vi "Data2Stats.vi"(0 "CMD Step":dbl format="%#_13g", 7 "DataIn":string[][](array[string]), 11 "DesiredParameters":T1) -> (8 "StatsOut":string[][](array[string]))   [LabVIEW 2013]
uses:
  TypeDef/Command Cluster.ctl
  <vilib>/Analysis/NI_AALBase.lvlib
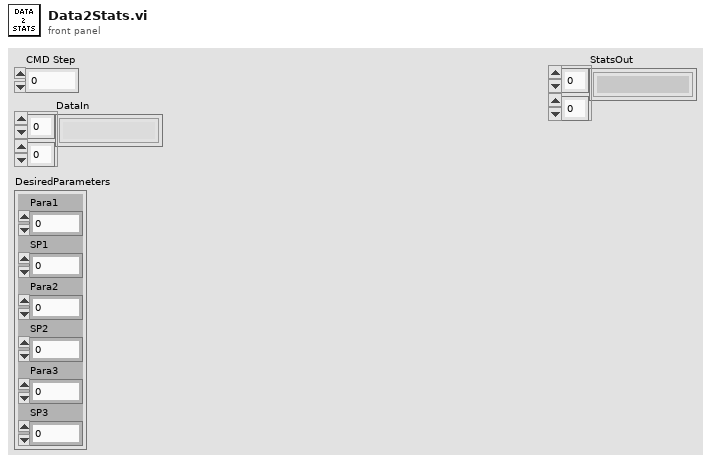
[diagram p1: front panel]
types:
  T1 = typedef "Command Cluster.ctl" = cluster{"Para1":i32, "SP1":dbl, "Para2":i32, "SP2":dbl, "Para3":i32, "SP3":dbl}
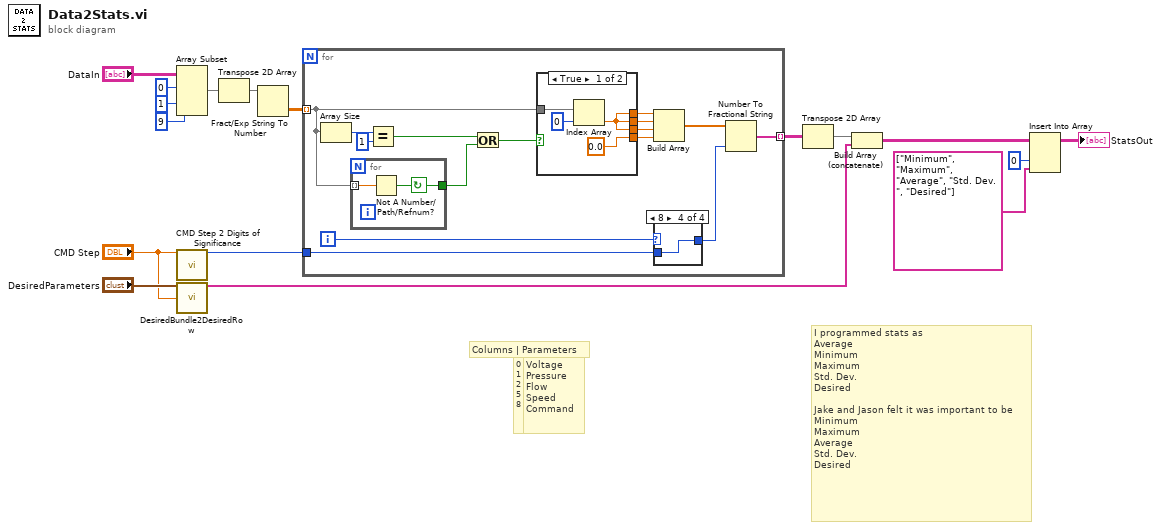
[diagram p0: block diagram]
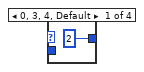
[diagram p2: hidden frame]
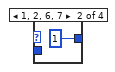
[diagram p3: hidden frame]
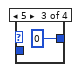
[diagram p4: hidden frame]
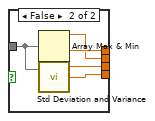
[diagram p5: hidden frame]
diagram:
  # "I programmed stats as\nAverage\nMinimum\nMaximum\nStd. Dev.\nDesired\n\nJake and Jason felt it was important to be\nMinimum\nMaximum\nAverage\nStd. Dev.\nDesired"
  # "Columns | Parameters"
  # "0\n1\n2\n5\n8"
  # "Voltage\nPressure\nFlow\nSpeed\nCommand"
  n1 = Array Subset(array="DataIn", index (row)=0 ("index"), index (col)=1 ("index"), length (col)=9 ("length")) -> (w13:string[][])  [unwired: 1 in]
  n2 = call "CMD Step 2 Digits of Significance.vi"("CMD Step"="CMD Step") -> ("Digits of Significance"=w2:i32)  [unwired: 14 in]
  n3 = call "DesiredBundle2DesiredRow.vi"("DesiredParameters"="DesiredParameters", "CMD Step"="CMD Step") -> ("DesiredStatRow"=w3:string[])  [unwired: 13 in]
  n4 = Transpose 2D Array(2D array=w13) -> (transposed array=w12:string[][])
  n5 = Fract/Exp String To Number(string=w12) -> (number=w11:dbl[][])  [unwired: 3 in, 1 out]
  n6 = for {
    tunnel: w11 -> [w21] mode=indexing
    tunnel: [w25] -> w5 mode=indexing
    tunnel: w2 -> [w22]
    i -> [w23]
    n7 = Array Size(array=w21) -> (size(s)=w28:i32)
    n8 = for {
      tunnel: w21 -> [w34] mode=indexing
      tunnel: [w33] -> w20
      stop <- w33 continue-if-true
      n9 = Not A Number/Path/Refnum?(number/path/refnum=w34) -> (NaN/Path/Refnum?=w33:bool)
    }
    n10 = Equal?(x=w28, y=1) -> (x = y?=w19:bool)
    n11 = Or(x=w19, y=w20) -> (x .or. y?=w18:bool)
    n12 = case shown="True" w18 {
      tunnel: [w40 w45] -> w32
      tunnel: [w40 w44] -> w31
      tunnel: [w40 w43] -> w30
      tunnel: [0.0 ("standard deviation") w47] -> w29
      tunnel: w21 -> [w42 w46]
      frame True {
        n13 = Index Array(array=w42, index=0) -> (element=w40:dbl)
      }
      frame False {
        n14 = Array Max & Min(array=w46) -> (max value=w44:dbl, min value=w45:dbl)  [unwired: 2 out]
        n15 = call <vilib>:"Std Deviation and Variance.vi"("X"=w46) -> ("mean"=w43:dbl, "standard deviation"=w47:dbl)  [unwired: 1 in, 1 out]
      }
    }
    n16 = Build Array(w32, w31, w30, w29) -> (w26:dbl[])
    n17 = case shown="8" w23 {
      tunnel: [2 1 0 w38] -> w24
      tunnel: w22 -> [_ _ _ w38]
      frame 0, 3, 4, Default {
      }
      frame 1, 2, 6, 7 {
      }
      frame 5 {
      }
      frame 8 {
      }
    }
    n18 = Number To Fractional String(number=w26, precision (6)=w24) -> (F-format string=w25:string[])  [unwired: 2 in]
  }
  n19 = Transpose 2D Array(2D array=w5) -> (transposed array=w10:string[][])
  n20 = Build Array (concatenate)(w10, w3) -> (w9:string[][])
  n21 = Insert Into Array(array=w9, index (col)=0 ("disabled index (col)"), new element=string[] ["Minimum", "Maximum", "Average", "Std. Dev.", "Desired"]) -> (→"StatsOut":string[][])  [unwired: 1 in]
